vi "Delete empty header content.vi"(8 "error in (no error)":errorcluster, 11 "Save Image in":refnum<class "Save Image.lvclass">) -> (0 "error out":errorcluster, 3 "Save Image out":refnum<class "Save Image.lvclass">)   [LabVIEW 2018, in "Save Image.lvclass"]
uses:
  Save Image.lvclass
  Save Image.lvclass/Save Image.ctl
  Header/Header.lvclass
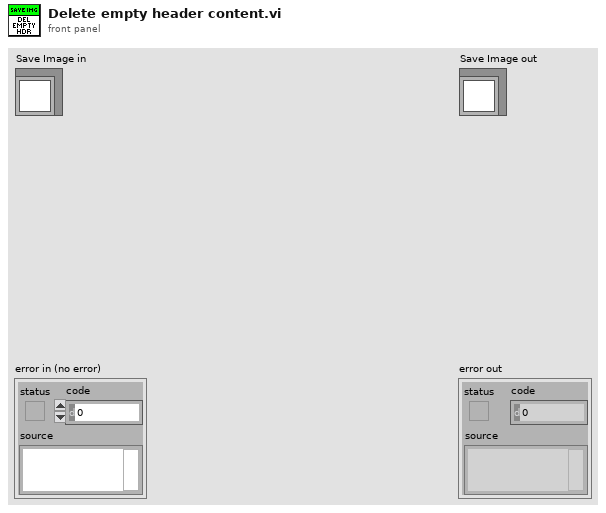
[diagram p1: front panel]
types:
  T1 = cluster{"Image Path":string, "Image Name":string, "Image Delays":string[]}
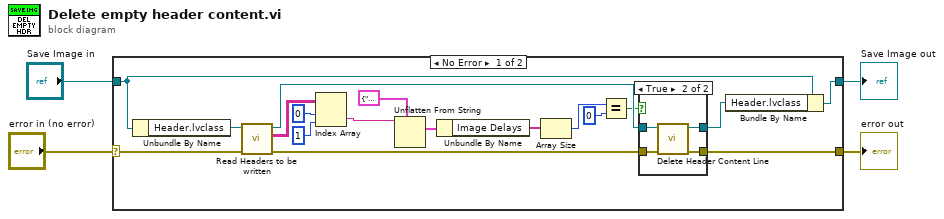
[diagram p0: block diagram]
diagram:
  n1 = case shown="No Error" "error in (no error)" {
    selector: "error in (no error)" -> [w20 w30]
    tunnel: [w16 w30] -> w3
    tunnel: [w14 w29] -> w1
    tunnel: "Save Image in" -> [w15 w29]
    frame No Error {
      n2 = Unbundle By Name(w15) -> ("Header.lvclass"=w19:refnum<class "Header.lvclass">)
      n3 = call "Read Headers to be written.vi"("error in (no error)"=w20, "Header in"=w19) -> ("error out"=w17:errorcluster, "Headers to be written"=w22:string[][], "Header out"=w18:refnum<class "Header.lvclass">)  [unwired: 7 in]
      n4 = Index Array(array=w22, index (row)=0, index (col)=1) -> (element=w10:string)
      n5 = Unflatten From String(type=T1 {"Image Path"="", "Image Name"="", "Image Delays"=[]} ("Image Delays Settings"), binary string=w10) -> (value=w9:T1)  [unwired: 3 in, 2 out]
      n6 = Unbundle By Name(w9) -> ("Image Delays"=w8:string[])
      n7 = Array Size(array=w8) -> (size(s)=w7:i32)
      n8 = Equal?(x=w7, y=0) -> (x = y?=w5:bool)
      n9 = case shown="True" w5 {
        tunnel: w18 -> [w24 w28]
        tunnel: w17 -> [w23 w27]
        tunnel: [w23 w26] -> w16
        tunnel: [w24 w25] -> w13
        frame False {
        }
        frame True {
          n10 = call "Delete Header Content Line.vi"("error in (no error)"=w27, "Header in"=w28) -> ("error out"=w26:errorcluster, "Header out"=w25:refnum<class "Header.lvclass">)  [unwired: 8 in]
        }
      }
      n11 = Bundle By Name(cluster=w15, "Header.lvclass"=w13) -> (w14:refnum<class "Save Image.lvclass">)
    }
    frame Error {
    }
  }
  "error out" <- w3
  "Save Image out" <- w1
